vi "Data Update.vi"(8 "error in (no error)":errorcluster, 10 "Data":cluster{"EDR":dbl, "Pulse":u8}, 11 "Controller in":refnum<class "Controller.lvclass">) -> (0 "error out":errorcluster, 3 "Controller out":refnum<class "Controller.lvclass">)   [LabVIEW 2011, in "Controller.lvclass"]
uses:
  Controller.lvclass
  Controller.lvclass/Controller.ctl
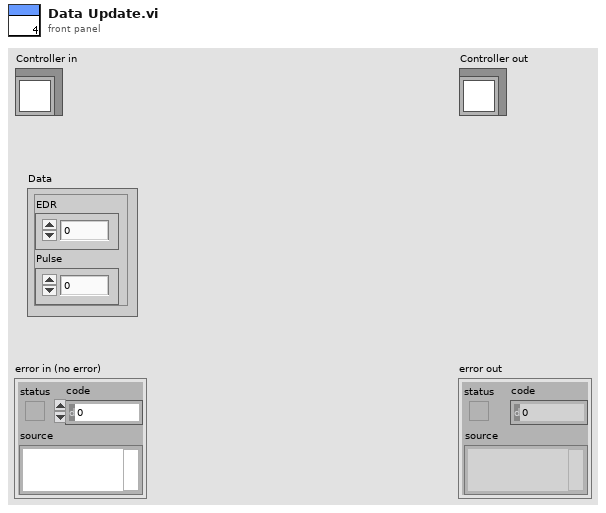
[diagram p1: front panel]
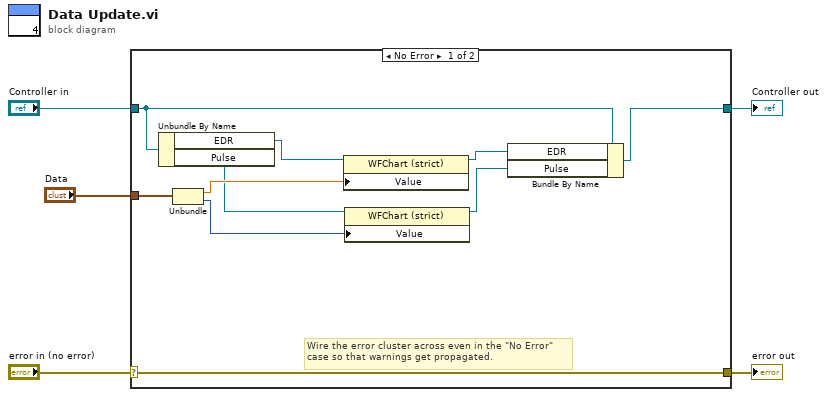
[diagram p0: block diagram]
diagram:
  n1 = case shown="No Error" "error in (no error)" {
    selector: "error in (no error)" -> [w15 w17]
    tunnel: [w15 w17] -> w4
    tunnel: [w6 w16] -> w2
    tunnel: "Controller in" -> [w7 w16]
    tunnel: "Data" -> [w14 _]
    frame No Error {
      # "Wire the error cluster across even in the \"No Error\"\ncase so that warnings get propagated."
      n2 = Unbundle By Name(w7) -> ("EDR"=w13:refnum<vi>, "Pulse"=w11:refnum<vi>)
      n3 = Unbundle(w14) -> ("EDR"=w12:dbl, "Pulse"=w10:u8)
      n4 = property class="WFChart (strict)"(reference=w13, "Value"=w12) -> (reference out=w9:refnum<vi>)  [unwired: 1 in, 1 out]
      n5 = property class="WFChart (strict)"(reference=w11, "Value"=w10) -> (reference out=w8:refnum<vi>)  [unwired: 1 in, 1 out]
      n6 = Bundle By Name(cluster=w7, "EDR"=w9, "Pulse"=w8) -> (w6:refnum<class "Controller.lvclass">)
    }
    frame Error {
    }
  }
  "error out" <- w4
  "Controller out" <- w2
